vi "Variable@RPopLPush__Parameter.vi"(1 "ParamterIn":string) -> (0 "ParamterOut":string)   [LabVIEW 2020]
panel:
  in  "Section":string(combo)
  in  "VarPush":string(combo)
  in  "VarPop":string(combo)
  in  "Confirm":bool
  # "Variable@RPopLPush $VariablePOP,$VariablePUSH(,$Section)"
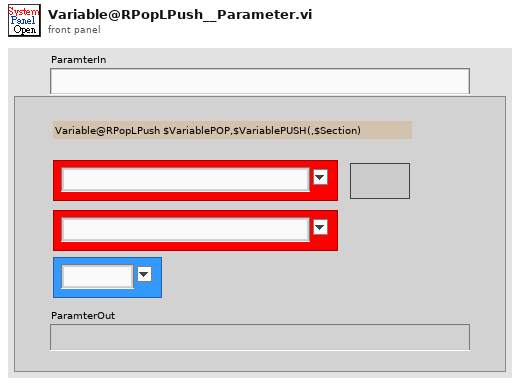
[diagram p1: front panel]
types:
  T1 = enum16{"Get", "Init", "Set", "Delete", "GetElement", "Inc", "Dec", "ReName"}
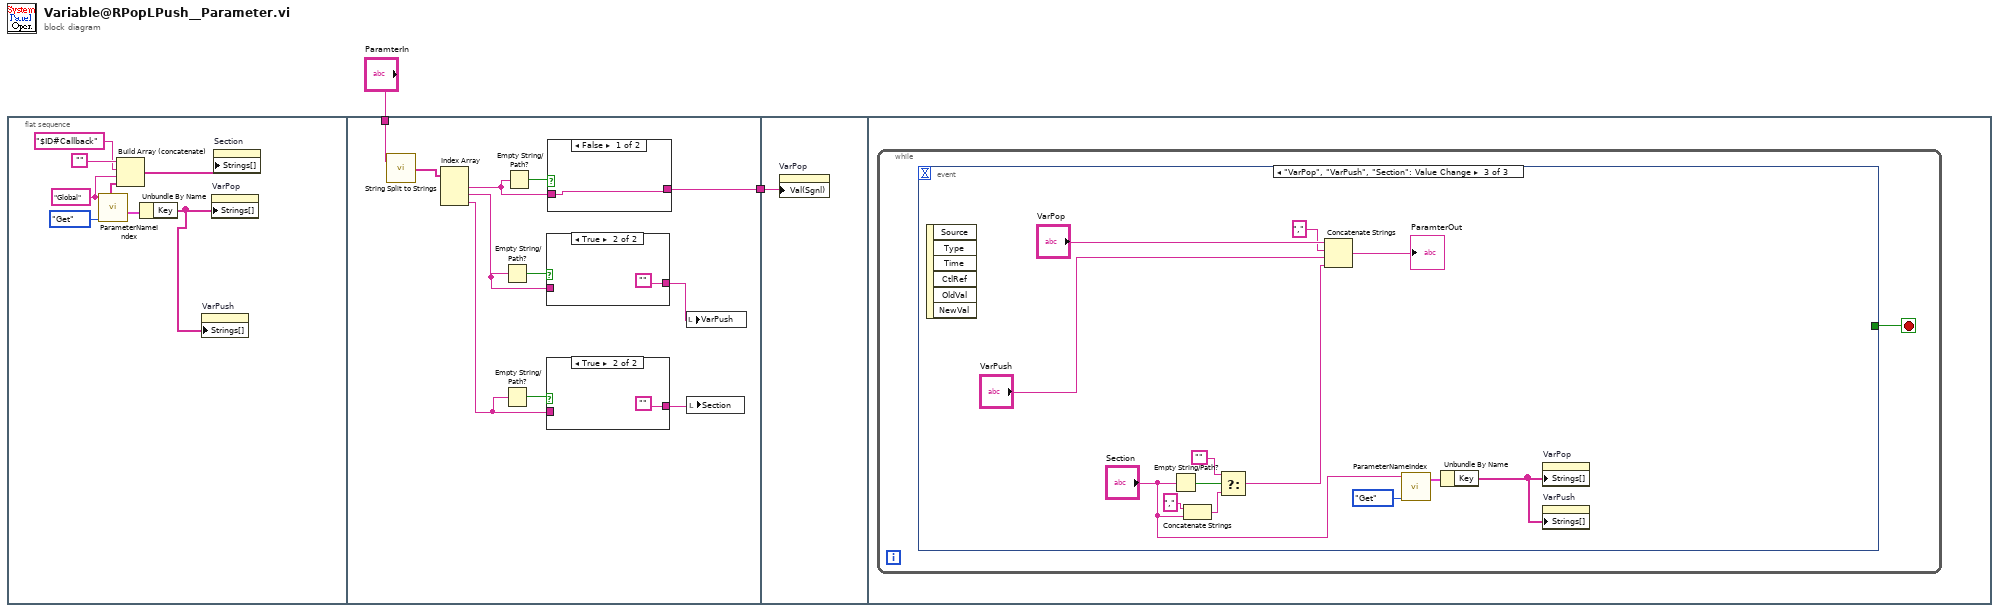
[diagram p0: block diagram]
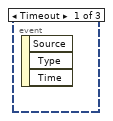
[diagram p5: hidden frame]
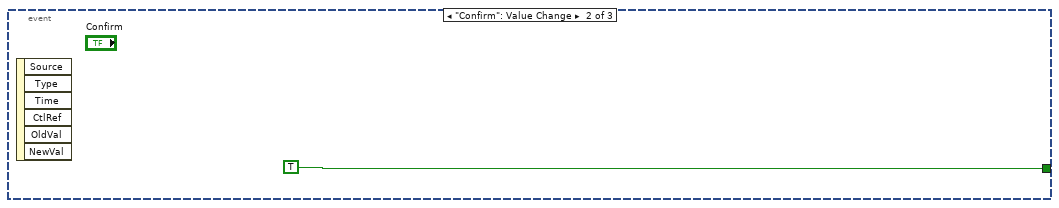
[diagram p6: hidden frame]
diagram:
  n1 = flat-sequence {
    tunnel: "ParamterIn" -> [w17]
    tunnel: [w19] -> w1
    tunnel: w1 -> [w28]
    frame #0 {
      w5 = "Global" ("VariableSection")
      n2 = call "ParameterNameIndex.vi"("OP"=T1."Get", "VariableSection"=w5) -> ("GlobalKeyValue"=w10:cluster{"Key":string[], "Value":string[]}, "SectionList"=w6:string[])  [unwired: 3 in, 5 out]
      n3 = Build Array (concatenate)("", "$ID#Callback" ("VariableSection"), w5, w6) -> (w4:string[])
      n4 = Unbundle By Name(w10) -> ("Key"=w8:string[])
      n5 = property on="VarPush" class="CmbBox"("Strings[]"=w8) -> ()  [unwired: 2 in, 2 out]
      n6 = property on="VarPop" class="CmbBox"("Strings[]"=w8) -> ()  [unwired: 2 in, 2 out]
      n7 = property on="Section" class="CmbBox"("Strings[]"=w4) -> ()  [unwired: 2 in, 2 out]
    }
    frame #1 {
      n8 = call "String Split to Strings.vi"("String"=w17) -> ("Array"=w16:string[])  [unwired: 1 in]
      n9 = Index Array(array=w16) -> (element #1=w15:string, element #2=w14:string, element #3=w12:string)  [unwired: 3 in]
      n10 = Empty String/Path?(string/path=w14) -> (empty?=w20:bool)
      n11 = Empty String/Path?(string/path=w12) -> (empty?=w13:bool)
      n12 = Empty String/Path?(string/path=w15) -> (empty?=w21:bool)
      n13 = case shown="True" w20 {
        tunnel: w14 -> [w24 _]
        tunnel: [w24 ""] -> w18
        frame False {
        }
        frame True {
        }
      }
      n14 = case shown="True" w13 {
        tunnel: w12 -> [w22 _]
        tunnel: [w22 ""] -> w11
        frame False {
        }
        frame True {
        }
      }
      n15 = case shown="False" w21 {
        tunnel: w15 -> [w26 w27]
        tunnel: [w26 w27] -> w19
        frame False {
        }
        frame True {
        }
      }
      n16 = local write "VarPush"(w18) -> ()
      n17 = local write "Section"(w11) -> ()
    }
    frame #2 {
      n18 = property on="VarPop" class="CmbBox"("Val(Sgnl)"=w28) -> ()  [unwired: 2 in, 2 out]
    }
    frame #3 {
      n19 = while {
        stop <- w29 stop-if-true
        n20 = event shown="[2] \"VarPop\", \"VarPush\", \"Section\": Value Change" {
          selector: _ -> [_ _ _]
          dyn-events: _ -> [_ _ _]
          timeout: _ -> [_ _ _]
          tunnel: [_ TRUE _] -> w29
          event Timeout {
            n21 = event-data() -> ()  [unwired: 1 in, 3 out]
          }
          event "Confirm": Value Change {
            n22 = event-data() -> ()  [unwired: 1 in, 6 out]
          }
          event "VarPop", "VarPush", "Section": Value Change {
            n23 = event-data() -> ()  [unwired: 1 in, 6 out]
            n24 = Empty String/Path?(string/path="Section") -> (empty?=w39:bool)
            n25 = Concatenate Strings("," ("string"), "Section") -> (w40:string)
            n26 = Select(t="", s=w39, f=w40) -> (s? t:f=w37:string)
            n27 = Concatenate Strings("VarPop", "," ("string"), "VarPush", w37) -> (→"ParamterOut":string)
            n28 = call "ParameterNameIndex.vi"("OP"=T1."Get", "VariableSection"="Section") -> ("SectionKeyValue"=w32:cluster{"Key":string[], "Value":string[]})  [unwired: 3 in, 6 out]
            n29 = Unbundle By Name(w32) -> ("Key"=w34:string[])
            n30 = property on="VarPop" class="CmbBox"("Strings[]"=w34) -> ()  [unwired: 2 in, 2 out]
            n31 = property on="VarPush" class="CmbBox"("Strings[]"=w34) -> ()  [unwired: 2 in, 2 out]
          }
        }
      }
    }
  }
